vi "LSCI332ReadCalFile.vi"(0 "Start path":path=path "" caption="Répertoire Initial", 11 "error in":errorcluster) -> (2 "No Courbe":u32=21 min=21 max=60 step=1, 3 "Nom":string="CourbeTest", 4 "No de série":string="Standard", 6 "Coefficient":u16(ring)=2 items=["Faites un choix", "négatif", "positif"], 10 "Table":string[][](table) caption="Table de Calibration", 13 "TLim":dbl=475.0 caption="T° de Contrôle Max (K)", 14 "Format":u16(ring)=2 items=["Faites un choix", "mV/K", "V/K", "Ohm/K", "log Ohm/K", "log Ohm/log K"], 15 "error out":errorcluster)   [LabVIEW 2019]
doc: "Ce Vi ouvre un fichier texte de calibration et retourne l'entête et les points points de calibration qui y sont sauvegardés"
panel:
  # "+5"
  # "+10"
  # "+15"
  # "+20"
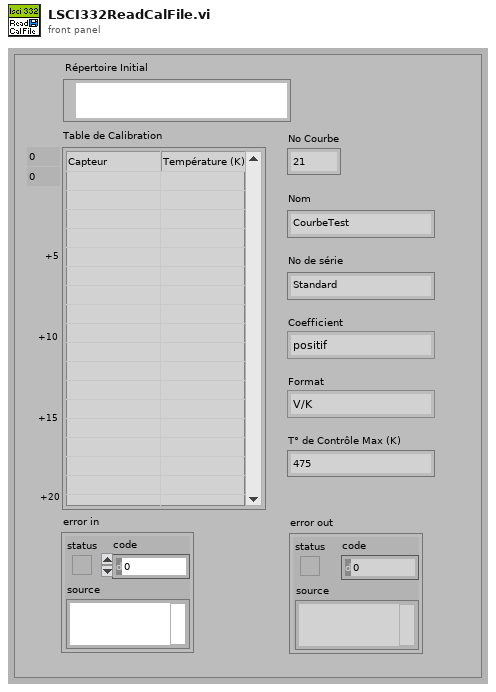
[diagram p1: front panel]
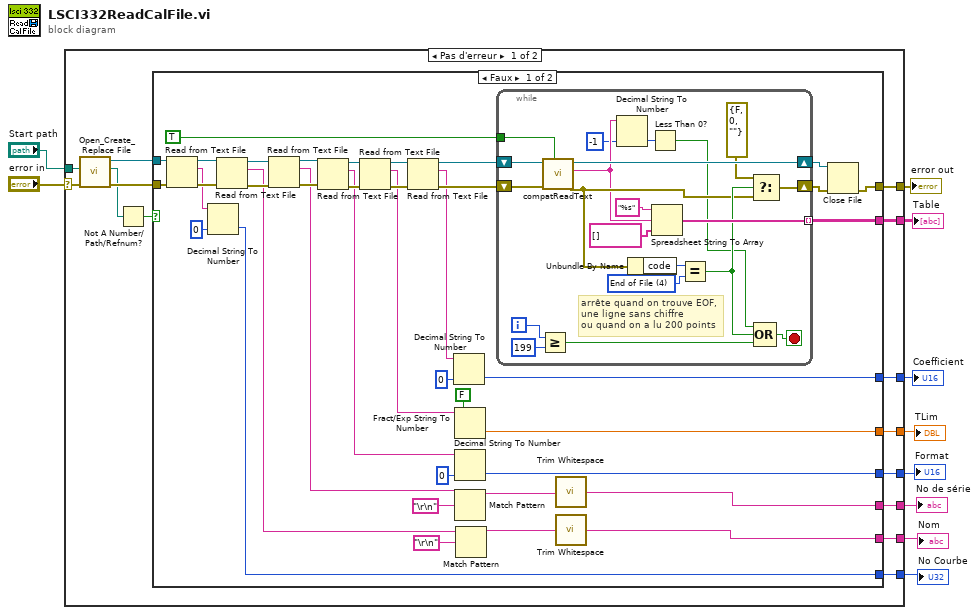
[diagram p0: block diagram]
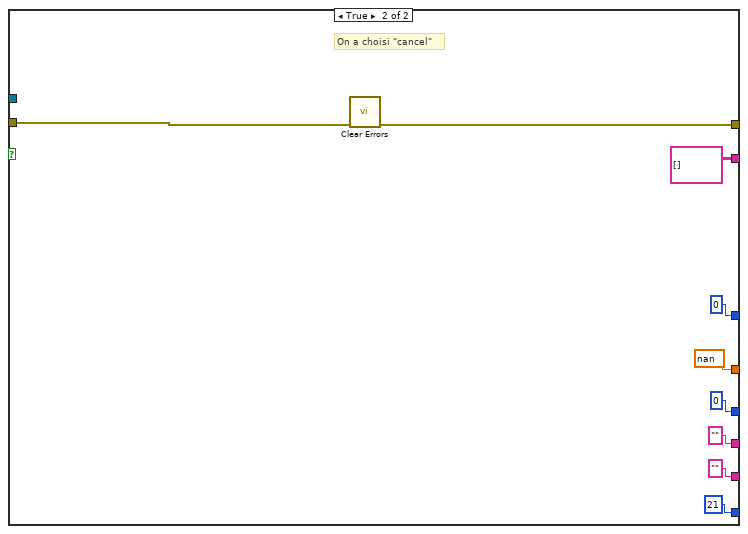
[diagram p2: hidden frame]
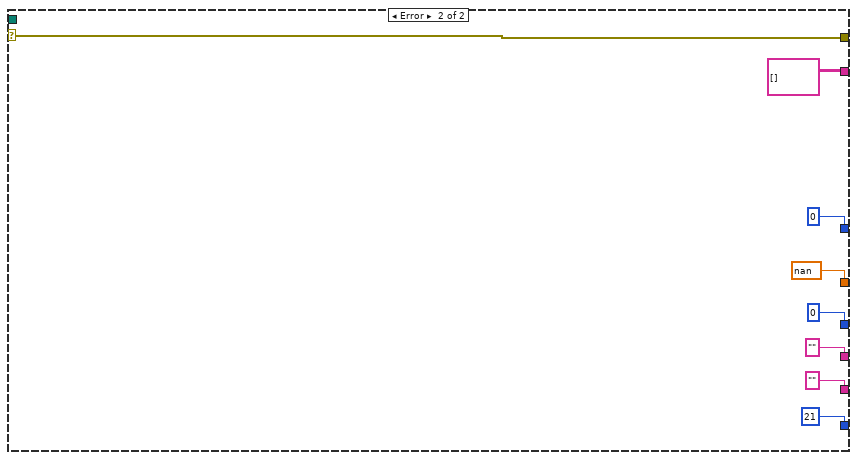
[diagram p3: hidden frame]
diagram:
  n1 = case shown="Pas d'erreur" "error in" {
    selector: "error in" -> [w22 w101]
    tunnel: [w21 w101] -> w9
    tunnel: "Start path" -> [w20 _]
    tunnel: [w17 string[][] []] -> w7
    tunnel: [w16 u32 21] -> w6
    tunnel: [w15 ""] -> w5
    tunnel: [w14 ""] -> w4
    tunnel: [w13 u16 0] -> w3
    tunnel: [w12 nan] -> w2
    tunnel: [w11 u16 0] -> w1
    frame No Error {
      n2 = call <vilib>:"Open_Create_Replace File.vi"("error in (no error)"=w22, "start path  (Not A Path)"=w20) -> ("error out"=w23:errorcluster, "new file path"=w19:path, "refnum"=w24:refnum<file>)  [unwired: 6 in, 1 out]
      n3 = Not A Number/Path/Refnum?(number/path/refnum=w19) -> (NaN/Path/Refnum?=w18:bool)
      n4 = case shown="Faux" w18 {
        tunnel: w24 -> [w63 _]
        tunnel: w23 -> [w62 w93]
        tunnel: [w43 w92] -> w21
        tunnel: [w37 string[][] []] -> w17
        tunnel: [w36 u32 21] -> w16
        tunnel: [w32 ""] -> w15
        tunnel: [w25 ""] -> w14
        tunnel: [w35 u16 0] -> w13
        tunnel: [w34 nan] -> w12
        tunnel: [w33 u16 0] -> w11
        frame False {
          n5 = Read from Text File(file (use dialog)=w63, error in=w62) -> (refnum out=w48:refnum<file>, text=w49:string, error out=w61:errorcluster)  [unwired: 2 in, 1 out]
          n6 = Decimal String To Number(string=w49, default (0L)=u32 0 ("default (0 I32)")) -> (number=w36:u32)  [unwired: 1 in, 1 out]
          n7 = Read from Text File(file (use dialog)=w48, error in=w61) -> (refnum out=w60:refnum<file>, text=w30:string, error out=w59:errorcluster)  [unwired: 2 in, 1 out]
          n8 = Read from Text File(file (use dialog)=w60, error in=w59) -> (refnum out=w58:refnum<file>, text=w27:string, error out=w57:errorcluster)  [unwired: 2 in, 1 out]
          n9 = Read from Text File(file (use dialog)=w58, error in=w57) -> (refnum out=w56:refnum<file>, text=w47:string, error out=w55:errorcluster)  [unwired: 2 in, 1 out]
          n10 = Read from Text File(file (use dialog)=w56, error in=w55) -> (refnum out=w53:refnum<file>, text=w45:string, error out=w54:errorcluster)  [unwired: 2 in, 1 out]
          n11 = Read from Text File(file (use dialog)=w53, error in=w54) -> (refnum out=w52:refnum<file>, text=w46:string, error out=w51:errorcluster)  [unwired: 2 in, 1 out]
          n12 = Decimal String To Number(string=w46, default (0L)=u16 0 ("default (0 I32)")) -> (number=w35:u16)  [unwired: 1 in, 1 out]
          n13 = Fract/Exp String To Number(use system decimal point (T)=FALSE, string=w45) -> (number=w34:dbl)  [unwired: 2 in, 1 out]
          n14 = Decimal String To Number(string=w47, default (0L)=u16 0 ("default (0 I32)")) -> (number=w33:u16)  [unwired: 1 in, 1 out]
          n15 = Match Pattern(string=w27, regular expression="\r\n") -> (before substring=w26:string)  [unwired: 1 in, 3 out]
          n16 = Match Pattern(string=w30, regular expression="\r\n") -> (before substring=w29:string)  [unwired: 1 in, 3 out]
          n17 = while {
            shift-right: [w82] -> w38
            shift-left: w52 -> [w84]
            shift-right: [w71] -> w50
            shift-left: w51 -> [w83]
            tunnel: [w75] -> w37 mode=indexing
            tunnel: TRUE -> [w76]
            i -> [w80]
            stop <- w78 stop-if-true
            w72 = 4 items=["No Error", "Manager Argument Error", "Memory Full", "Out of Zone", "End of File", "File Already Open", "Generic File IO Error", "File Not Found", "File Permission Error", "Disk Full", "Duplicate Path", "Too Many Files Open", "Not Enabled", "Resource File Not Found", "Cannot Add Resource", "Resource Not Found", "Image Not Found", "Image Memory Error", "Pen Does Not Exist", "Config Bad Type", "Config Token Not Found", "Config Parse Error", "Config Memory Error", "Bad External Code Format", "Bad External Code Offset", "External Code Not Present", "Null Window", "Destroy Window Mixup", "Null Menu", "Print Aborted", "Bad Print Record", "Print Driver Error", "Windows Error During Print", "Memory Error During Print", "Print Dialog Error", "Generic Print Error", "Invalid Device Refnum", "Device Not Found", "Device Parameter Error", "Device Unit Error", "Can't Open Device", "Device Call Aborted", "Generic Error", "Cancelled By User", "Object ID Too Low", "Object ID Too High", "Object Not In Heap", "Unknown Heap", "Bad DefProc ID", "DefProc Not In Table", "Message Out Of Range", "Null Method", "Unknown Message", "Manager Call Not Supported"]
            # "arrête quand on trouve EOF,\nune ligne sans chiffre\nou quand on a lu 200 points"
            n18 = Greater Or Equal?(x=w80, y=199) -> (x >= y?=w77:bool)
            n19 = call <vilib>:"compatReadText.vi"("line mode (F)"=w76, "error in"=w83, "refnum"=w84) -> ("error out"=w69:errorcluster, "data"=w67:string, "dup refnum"=w82:refnum<file>)  [unwired: 6 in]
            n20 = Decimal String To Number(string=w67, default (0L)=-1 ("default (0 I32)")) -> (number=w65:i32)  [unwired: 1 in, 1 out]
            n21 = Unbundle By Name(w69) -> ("code"=w73:i32)
            n22 = Less Than 0?(x=w65) -> (x < 0?=w64:bool)
            n23 = Spreadsheet String To Array(format string="%s", spreadsheet string=w67, array type (2D Dbl)=string[] []) -> (array=w75:string[])  [unwired: 1 in]
            n24 = Equal?(x=w73, y=w72) -> (x = y?=w70:bool)
            n25 = Select(t=errorcluster {"status"=FALSE, "code"=0, "source"=""} ("error out"), s=w70, f=w69) -> (s? t:f=w71:errorcluster)
            n26 = Compound Arithmetic op=OR(w64, w70, w77) -> (w78:bool)
          }
          n27 = call <vilib>:"Trim Whitespace.vi"("string"=w26) -> ("trimmed string"=w25:string)  [unwired: 1 in]
          n28 = call <vilib>:"Trim Whitespace.vi"("string"=w29) -> ("trimmed string"=w32:string)  [unwired: 1 in]
          n29 = Close File(refnum=w38, error in=w50) -> (error out=w43:errorcluster)  [unwired: 1 out]
        }
        frame True {
          # "On a choisi \"cancel\""
          n30 = call <vilib>:"Clear Errors.vi"("error in (no error)"=w93) -> ("error out"=w92:errorcluster)  [unwired: 5 in, 1 out]
        }
      }
    }
    frame Error {
    }
  }
  "error out" <- w9
  "Table" <- w7
  "Nom" <- w5
  "No de série" <- w4
  "No Courbe" <- w6
  "Format" <- w1
  "TLim" <- w2
  "Coefficient" <- w3
